vi "Add (String).vi"(8 "error in (no error)":errorcluster, 9 "Value":string, 10 "Name":string, 11 "Sequence Constants in":refnum<class "Sequence Constants.lvclass">) -> (0 "error out":errorcluster, 3 "Sequence Constants out":refnum<class "Sequence Constants.lvclass">)   [LabVIEW 2023, in "VolatusSeqConfig.lvlib" / "Sequence Constants.lvclass"]
uses:
  Sequence Constants.lvclass
  Sequence Constants.lvclass/Sequence Constants.ctl
  lv-cdm/CDM-Config/Config Element/Config Element.lvclass
  lv-cdm/CDM-Config/Value Type.ctl
  lv-cdm/CDM-Config/CDM-Config.lvlib
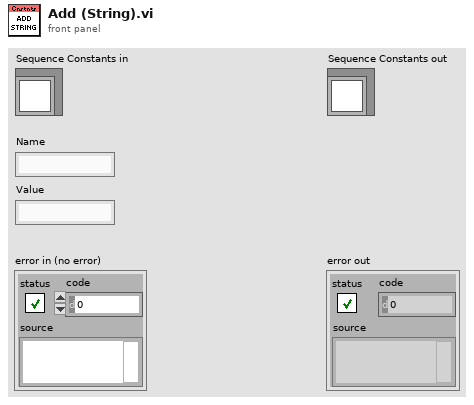
[diagram p1: front panel]
types:
  T1 = typedef "CDM-Config.lvlib/Value Type.ctl" = enum16{"String", "Number", "Bool", "Object", "Array"}
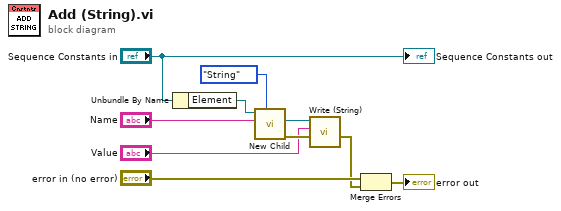
[diagram p0: block diagram]
diagram:
  n1 = Unbundle By Name("Sequence Constants in") -> ("Element"=w8:refnum<class "Config Element.lvclass">)
  n2 = call "New Child.vi"("Value Type (Object)"=Value_Type."String", "Child Name"="Name", "Config Element in"=w8) -> ("error out"=w5:errorcluster, "New Child"=w4:refnum<class "Config Element.lvclass">)  [unwired: 6 in, 1 out]
  n3 = call "Write (String).vi"("error in (no error)"=w5, "String Value"="Value", "Config Element in"=w4) -> ("error out"=w1:errorcluster)  [unwired: 7 in, 1 out]
  n4 = Merge Errors("error in (no error)", w1) -> (→"error out":errorcluster)
  "Sequence Constants out" <- "Sequence Constants in"
